vi "FindTreeKey_alt.vi"(8 "error in (no error)":errorcluster, 10 "Key":T3, 11 "Map":T4) -> (0 "error out":errorcluster, 1 "How rotated?":i8[](array[numeric]), 2 "DecisionRecord":T1, 3 "IsFound?":bool)   [LabVIEW 2020]
uses:
  controls/DecisionTree.ctl
  controls/Gameboard Data.ctl
  controls/DecisionTreeRecord.ctl
  controls/Player.ctl
  MakeSquare.vi
  Flatten2DArray.vi
  <vilib>/Utility/error.llb/Error Cluster From Error Code.vi
  GetAllIsometriesOf2DArray.vi
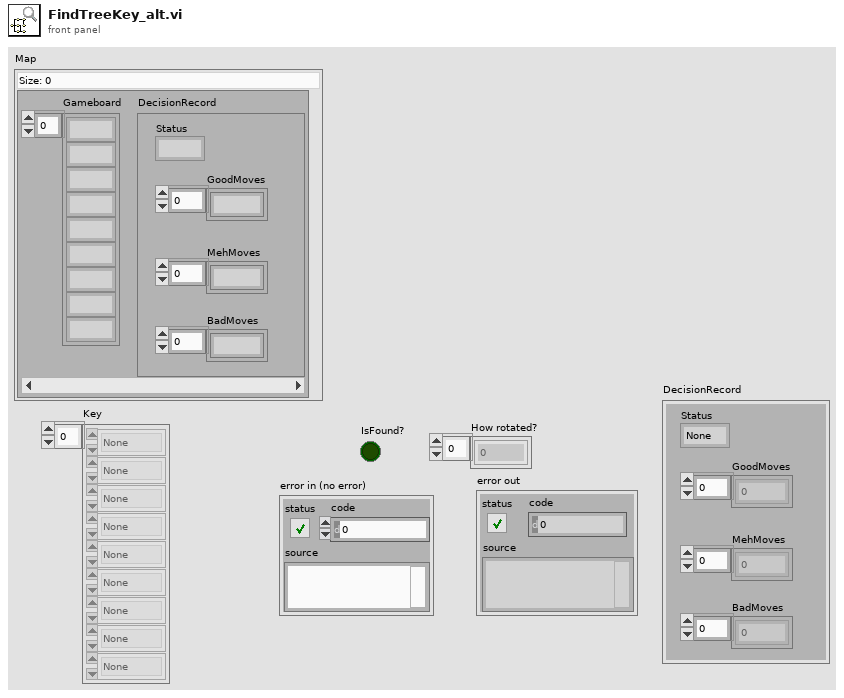
[diagram p1: front panel]
types:
  T1 = typedef "DecisionTreeRecord.ctl" = cluster{"Status":T2, "GoodMoves":i8[], "MehMoves":i8[], "BadMoves":i8[]}
  T2 = typedef "Player.ctl" = enum16{"None", "Player 1", "Player 2"}
  T3 = typedef "Gameboard Data.ctl" = enum16{"None", "Player 1", "Player 2"}[]
  T4 = typedef "DecisionTree.ctl" = map{T3, T1}
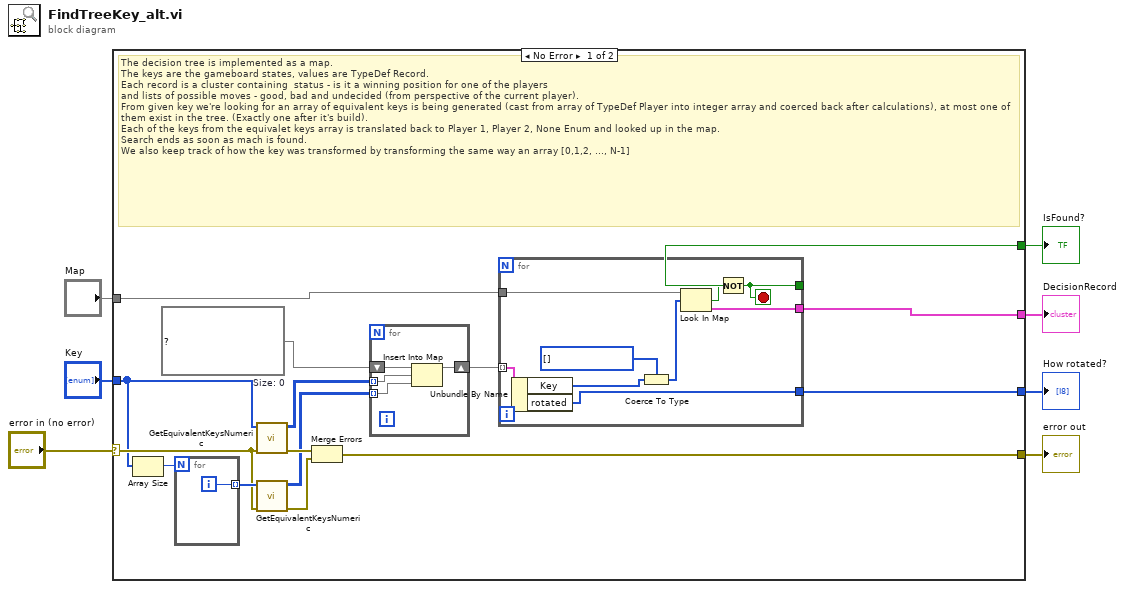
[diagram p0: block diagram]
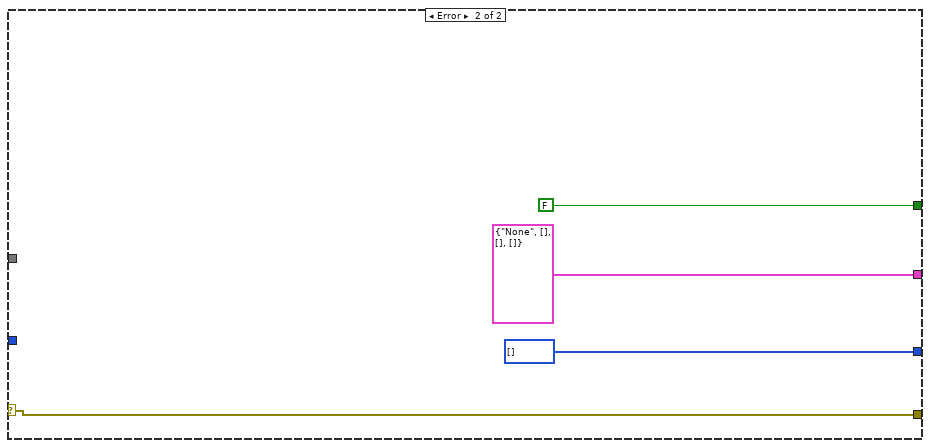
[diagram p2: hidden frame]
diagram:
  n1 = case shown="No Error" "error in (no error)" {
    selector: "error in (no error)" -> [w17 w40]
    tunnel: [w12 w40] -> w6
    tunnel: "Map" -> [w15 _]
    tunnel: "Key" -> [w13 _]
    tunnel: [w22 FALSE] -> w3
    tunnel: [w14 T1 {"Status"=enum."None", "GoodMoves"=[], "MehMoves"=[], "BadMoves"=[]} ("DecisionRecord")] -> w1
    tunnel: [w18 i8[] [] ("KeysEquivalenceClassNumeric")] -> w2
    frame No Error {
      w9 = map{i8[], i8[]} {}  # Size: 0
      # "The decision tree is implemented as a map. \nThe keys are the gameboard states, values are TypeDef Record.\nEach record is a cluster containing  status - is it a winning position for one of the players \nand lists of possible moves - good, bad and undecided (from perspective of the current player).\nFrom given key we're looking for an array of equivalent keys is being generated (cast from array of TypeDef Player into integer array and coerced back after calculations), at most one of them exist in the tree. (Exactly one after it's build).\nEach of the keys from the equivalet keys array is translated back to Player 1, Player 2, None Enum and looked up in the map. \nSearch ends as soon as mach is found.\nWe also keep track of how the key was transformed by transforming the same way an array [0,1,2, ..., N-1]"
      n2 = Array Size(array=w13) -> (size(s)=w20:i32)
      n3 = for {
        N: w20 -> [_]
        tunnel: [w36] -> w19 mode=indexing
        i -> [w36]
      }
      n4 = call "GetEquivalentKeysNumeric.vi"("error in (no error)"=w17, "KeyNumeric"=w13) -> ("error out"=w16:errorcluster, "KeysEquivalenceClassNumeric"=w11:i8[][])  [unwired: 8 in]
      n5 = call "GetEquivalentKeysNumeric.vi"("error in (no error)"=w17, "KeyNumeric"=w19) -> ("error out"=w21:errorcluster, "KeysEquivalenceClassNumeric"=w10:i8[][])  [unwired: 8 in]
      n6 = Merge Errors(w16, w21) -> (w12:errorcluster)
      n7 = for {
        tunnel: w11 -> [w26] mode=indexing
        tunnel: w10 -> [w25] mode=indexing
        shift-right: [w23] -> w8
        shift-left: w9 -> [w24]
        n8 = Insert Into Map(map in=w24, key=w26, value=w25) -> (map out=w23:map{i8[], i8[]})  [unwired: 2 out]
      }
      n9 = for {
        tunnel: [w30] -> w22
        tunnel: [w27] -> w18
        tunnel: w15 -> [w35]
        tunnel: [w34] -> w14
        tunnel: w8 -> [w29] mode=indexing
        stop <- w30 stop-if-true
        w31 = T2[] [] items=["None", "Player 1", "Player 2"] ("Array")
        n10 = Unbundle By Name(w29) -> ("Key"=w28:i8[], "rotated"=w27:i8[])
        n11 = Coerce To Type(0:w28, 1:w31) -> (2:w32:T2[])
        n12 = Look In Map(map=w35, key=w32) -> (key not found?=w33:bool, value=w34:T1)  [unwired: 1 in]
        n13 = Not(x=w33) -> (.not. x?=w30:bool)
      }
    }
    frame Error {
    }
  }
  "IsFound?" <- w3
  "DecisionRecord" <- w1
  "error out" <- w6
  "How rotated?" <- w2
